vi "Close SHV Connections.vi"(8 "error in (no error)":errorcluster, 11 "Samples in":refnum<class "Samples.lvclass">) -> (0 "error out":errorcluster, 3 "Samples out":refnum<class "Samples.lvclass">)   [LabVIEW 2015, in "AMS UI.lvlib" / "Samples.lvclass"]
uses:
  Samples.lvclass
  Samples.lvclass/Samples.ctl
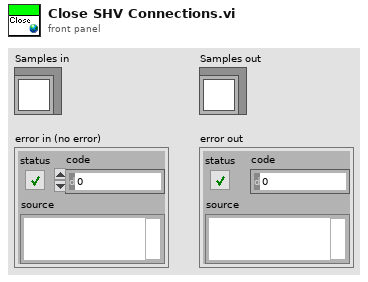
[diagram p1: front panel]
types:
  T1 = typedef "Sample Container.ctl" = cluster{"Sample In":refnum<k21>, "Sample Name":refnum<k21>, "Ti Cathode":refnum<k21>, "SampleQ":refnum<queue>}
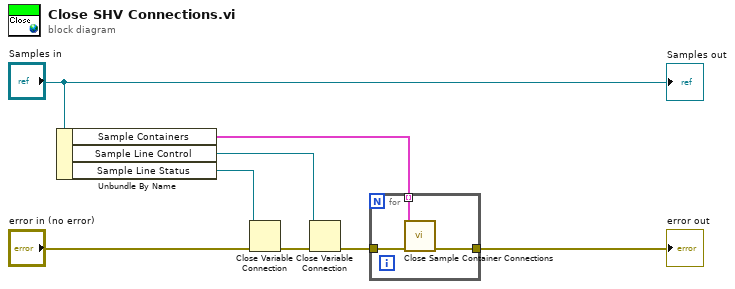
[diagram p0: block diagram]
diagram:
  n1 = Unbundle By Name("Samples in") -> ("Sample Containers"=w5:T1[], "Sample Line Control"=w8:refnum<k21>, "Sample Line Status"=w7:refnum<k21>)
  n2 = Close Variable Connection(8:"error in (no error)", 11:w7) -> (0:w3:errorcluster)
  n3 = Close Variable Connection(8:w3, 11:w8) -> (0:w2:errorcluster)
  n4 = for {
    tunnel: w5 -> [w10] mode=indexing
    tunnel: w2 -> [w11]
    tunnel: [w9] -> w4
    n5 = call "Close Sample Container Connections.vi"("error in (no error)"=w11, "Container in"=w10) -> ("error out"=w9:errorcluster)  [unwired: 8 in, 1 out]
  }
  "error out" <- w4
  "Samples out" <- "Samples in"
